vi "GetDescription.vi"(8 "error in (no error)":errorcluster) -> (0 "error out":errorcluster, 3 "text out":string)   [LabVIEW 2010, in "Licenses.lvlib"]
uses:
  Licenses.lvlib
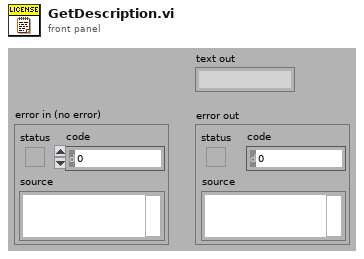
[diagram p1: front panel]
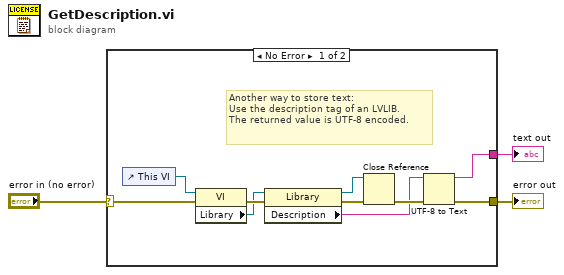
[diagram p0: block diagram]
diagram:
  n1 = case shown="No Error" "error in (no error)" {
    selector: "error in (no error)" -> [w5 w14]
    tunnel: [w13 w14] -> w3
    tunnel: [w10 _] -> w2
    frame No Error {
      # "Another way to store text:\nUse the description tag of an LVLIB.\nThe returned value is UTF-8 encoded."
      n2 = control-ref of="This VI"() -> (w4:refnum<vi>)
      n3 = property class="VI"(reference=w4, error in=w5) -> (error out=w7:errorcluster, "Library"=w6:refnum<vi>)  [unwired: 1 out]
      n4 = property class="Library"(reference=w6, error in=w7) -> (reference out=w9:refnum<vi>, error out=w11:errorcluster, "Description"=w8:string)
      n5 = Close Reference(reference=w9, error in (no error)=w11) -> (error out=w12:errorcluster)
      n6 = UTF-8 to Text(8:w12, 11:w8) -> (0:w13:errorcluster, 3:w10:string)
    }
    frame Error {
    }
  }
  "error out" <- w3
  "text out" <- w2
